vi "Extra_Commands.vi"(4 "offset (0)":i32, 5 "String to Search":string, 7 "Command":string) -> (0 "Offset Past Command":i32, 1 "Numeric Value":dbl format="%.2f", 2 "String Value":string, 3 "Command Found":bool)   [LabVIEW 2018]
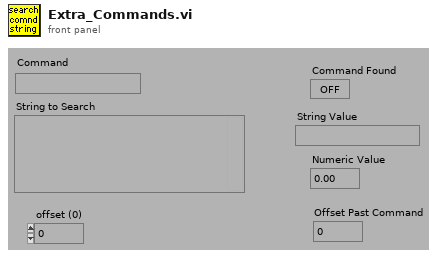
[diagram p1: front panel]
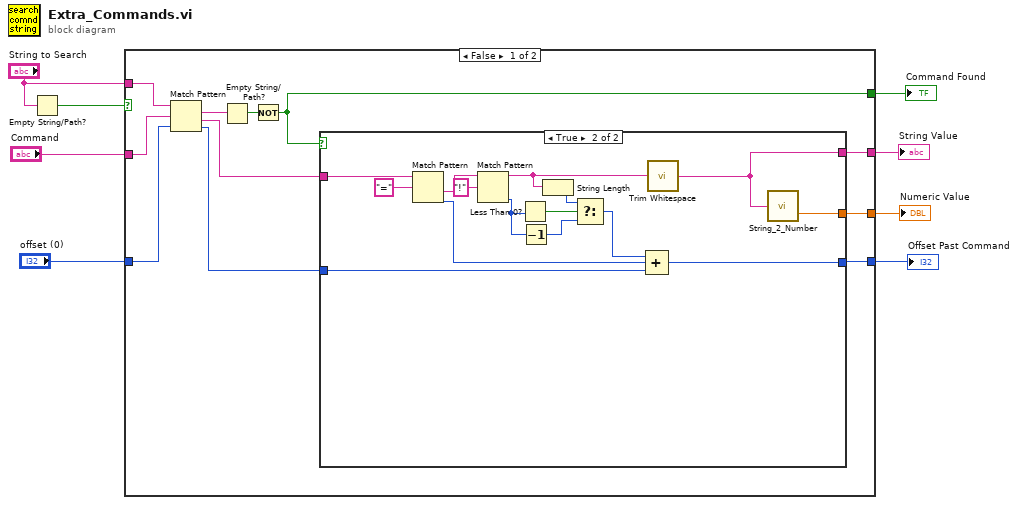
[diagram p0: block diagram]
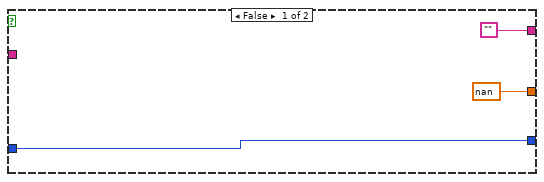
[diagram p2: hidden frame]
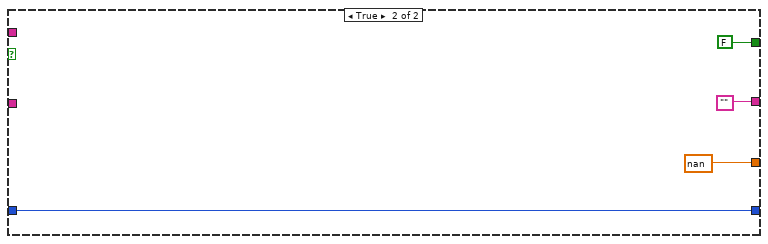
[diagram p3: hidden frame]
diagram:
  n1 = Empty String/Path?(string/path="String to Search") -> (empty?=w2:bool)
  n2 = case shown="False" w2 {
    tunnel: [w17 ""] -> w8
    tunnel: [w16 nan] -> w7
    tunnel: [w15 FALSE] -> w6
    tunnel: [w13 w38] -> w5
    tunnel: "offset (0)" -> [w12 w38]
    tunnel: "Command" -> [w11 _]
    tunnel: "String to Search" -> [w9 _]
    frame False {
      n3 = Match Pattern(string=w9, regular expression=w11, offset (0)=w12) -> (match substring=w19:string, after substring=w10:string, offset past match=w14:i32)  [unwired: 1 out]
      n4 = Empty String/Path?(string/path=w19) -> (empty?=w18:bool)
      n5 = Not(x=w18) -> (.not. x?=w15:bool)
      n6 = case shown="True" w15 {
        tunnel: ["" w25] -> w17
        tunnel: [nan w34] -> w16
        tunnel: w14 -> [w20 w24]
        tunnel: [w20 w32] -> w13
        tunnel: w10 -> [_ w23]
        frame False {
        }
        frame True {
          n7 = Match Pattern(string=w23, regular expression="=") -> (after substring=w35:string, offset past match=w33:i32)  [unwired: 3 out]
          n8 = Match Pattern(string=w35, regular expression="!") -> (before substring=w26:string, offset past match=w29:i32)  [unwired: 3 out]
          n9 = Less Than 0?(x=w29) -> (x < 0?=w31:bool)
          n10 = Decrement(x=w29) -> (x-1=w27:i32)
          n11 = String Length(string=w26) -> (length=w30:i32)
          n12 = Select(t=w30, s=w31, f=w27) -> (s? t:f=w28:i32)
          n13 = Compound Arithmetic op=ADD(w28, w33, w24) -> (w32:i32)
          n14 = call <vilib>:"Trim Whitespace.vi"("string"=w26) -> ("trimmed string"=w25:string)  [unwired: 1 in]
          n15 = call "String_2_Number.vi"("Value"=w25) -> ("Numeric"=w34:dbl)
        }
      }
    }
    frame True {
    }
  }
  "Command Found" <- w6
  "String Value" <- w8
  "Numeric Value" <- w7
  "Offset Past Command" <- w5
